vi "BRig_Host__Loop_Consumer_RunState__closedLoop_parseOutput2_cmd.vi"(11 "String":string) -> (2 "output_cmdList":u16[][](array[numeric]), 3 "output_cmdList":bool)   [LabVIEW 2014]
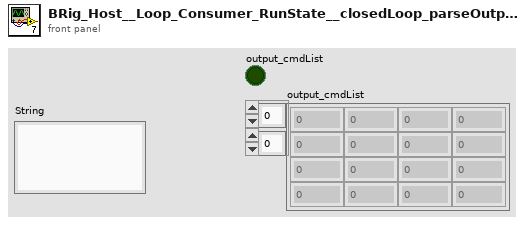
[diagram p1: front panel]
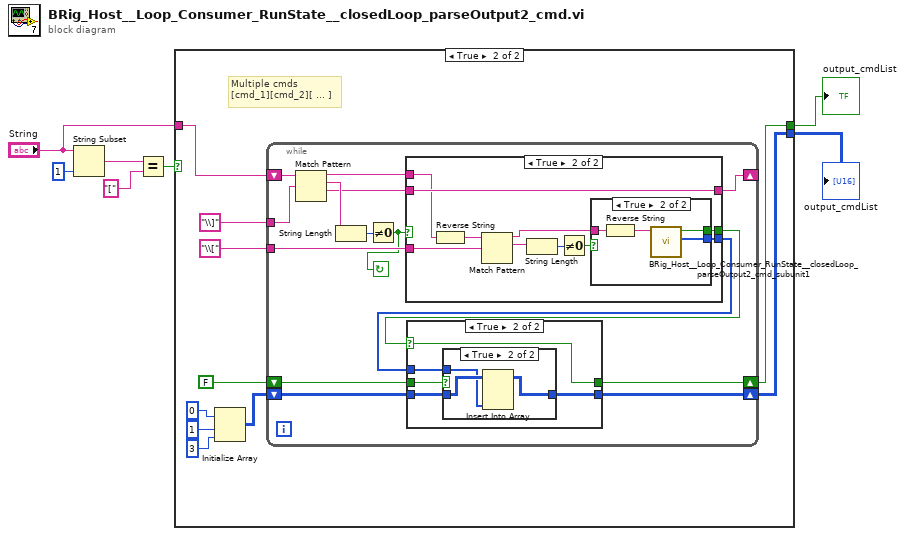
[diagram p0: block diagram]
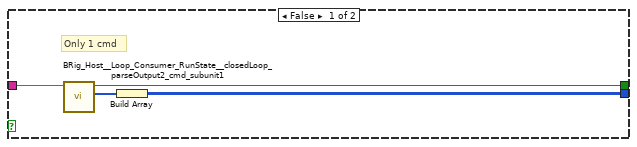
[diagram p2: hidden frame]
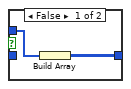
[diagram p4: hidden frame]
diagram:
  n1 = String Subset(string="String", length (rest)=1 ("length (rest)")) -> (substring=w6:string)  [unwired: 1 in]
  n2 = Equal?(x=w6, y="[") -> (x = y?=w5:bool)
  n3 = case shown="True" w5 {
    tunnel: "String" -> [w11 w21]
    tunnel: [w9 w15] -> w2
    tunnel: [w8 w14] -> w1
    frame False {
      # "Only 1 cmd"
      n4 = call "BRig_Host__Loop_Consumer_RunState__closedLoop_parseOutput2_cmd_subunit1.vi"("String"=w11) -> (2:"output_cmd"=w10:u16[], 3:"output_cmd"=w9:bool)  [unwired: 9 in]
      n5 = Build Array(w10) -> (w8:u16[][])
    }
    frame True {
      # "Multiple cmds\n[cmd_1][cmd_2][ ... ]"
      n6 = Initialize Array(u16 0, 1 ("dimension size"), 3 ("dimension size")) -> (w16:u16[][])
      n7 = while {
        shift-right: [w31] -> _
        shift-left: w21 -> [w36]
        shift-right: [w26] -> w15
        shift-left: FALSE -> [w28]
        shift-right: [w25] -> w14
        shift-left: w16 -> [w27]
        tunnel: "\\]" ("y") -> [w24]
        tunnel: "\\[" ("y") -> [w23]
        stop <- w22 continue-if-true
        n8 = Match Pattern(string=w36, regular expression=w24) -> (before substring=w32:string, match substring=w34:string, after substring=w33:string)  [unwired: 1 in, 1 out]
        n9 = String Length(string=w34) -> (length=w35:i32)
        n10 = Not Equal To 0?(x=w35) -> (x != 0?=w22:bool)
        n11 = case shown="True" w22 {
          tunnel: w33 -> [w49 w59]
          tunnel: w32 -> [_ w58]
          tunnel: [w49 w59] -> w31
          tunnel: [_ w52] -> w30
          tunnel: [_ w51] -> w29
          tunnel: w23 -> [_ w50]
          frame False {
          }
          frame True {
            n12 = Reverse String(1:w58) -> (0:w57:string)
            n13 = Match Pattern(string=w57, regular expression=w50) -> (before substring=w53:string, match substring=w55:string)  [unwired: 1 in, 2 out]
            n14 = String Length(string=w55) -> (length=w56:i32)
            n15 = Not Equal To 0?(x=w56) -> (x != 0?=w54:bool)
            n16 = case shown="True" w54 {
              tunnel: w53 -> [_ w63]
              tunnel: [_ w61] -> w52
              tunnel: [_ w60] -> w51
              frame False {
              }
              frame True {
                n17 = Reverse String(1:w63) -> (0:w62:string)
                n18 = call "BRig_Host__Loop_Consumer_RunState__closedLoop_parseOutput2_cmd_subunit1.vi"("String"=w62) -> (2:"output_cmd"=w61:u16[], 3:"output_cmd"=w60:bool)  [unwired: 9 in]
              }
            }
          }
        }
        n19 = case shown="True" w29 {
          selector: w29 -> [_ w39]
          tunnel: w30 -> [_ w41]
          tunnel: w28 -> [w38 w43]
          tunnel: w27 -> [w37 w42]
          tunnel: [w38 w39] -> w26
          tunnel: [w37 w40] -> w25
          frame False {
          }
          frame True {
            n20 = case shown="True" w43 {
              tunnel: w42 -> [_ w48]
              tunnel: w41 -> [w45 w47]
              tunnel: [w44 w46] -> w40
              frame False {
                n21 = Build Array(w45) -> (w44:u16[][])
              }
              frame True {
                n22 = Insert Into Array(array=w48, new element=w47) -> (w46:u16[][])  [unwired: 2 in]
              }
            }
          }
        }
      }
    }
  }
  "output_cmdList" <- w2
  "output_cmdList" <- w1
